vi "CreateClass.vi"(0 "ClassWriterGOOP300.lvclass":refnum<class "ClassWriterGOOP300.lvclass">, 1 "ProjectTreePosition(String or Project Item Ref)":variant, 2 "CreateClassData":T1, 5 "error in (no error)":errorcluster, 6 "KeepLvClassRefOpen(False)":bool, 7 "HeaderToApply (take from VIRef or /use 2D-8bit header, Ignored if not wired)":variant) -> (14 "ClassWriterGOOP300.lvclass":refnum<class "ClassWriterGOOP300.lvclass">, 15 "LVClassLibraryRefnum":refnum<vi>, 16 "TemplateVersionUsed":string, 19 "error out":errorcluster)   [LabVIEW 2020, in "ClassWriterGOOP300.lvclass"]
uses:
  <resource>/Framework/Providers/Open_GDS/ClassProviders/Provider_EndevoGOOP300/ClassWriterGOOP300_class/ClassWriterGOOP300.lvclass
  <resource>/Framework/Providers/Open_GDS/ClassProviders/Provider_BaseClassInterface/CreateClassData.ctl
  <resource>/Framework/Providers/Open_GDS/ClassProviders/Common/LvClass_class/GDSLvCLass_ClassSettingsType.ctl
  <resource>/Framework/Providers/Open_GDS/ClassProviders/Common/LvClass_class/GDSLvClass_PlugIn.ctl
  <resource>/Framework/Providers/Open_GDS/ClassProviders/Common/LvClass_class/GDSLvClass_PlugInTypes.ctl
  <resource>/Framework/Providers/Open_GDS/ClassProviders/Provider_EndevoGOOP400/EndevoG4ProviderName.ctl
  <resource>/Framework/Providers/Open_GDS/ClassProviders/Provider_EndevoGOOP300/EndevoProviderName.ctl
  <resource>/Framework/Providers/Open_GDS/ClassProviders/Provider_BaseClassInterface/ClassWriter_class/ClassWriter.lvclass
  <resource>/Framework/Providers/Open_GDS/ClassProviders/Provider_LvNativeClass/ClassWriterNative_class/ClassWriterNative.lvclass
  <resource>/Framework/Providers/Open_GDS/ClassProviders/Provider_EndevoGOOP400/ClassWriterGOOP400_class/ClassWriterGOOP400.lvclass
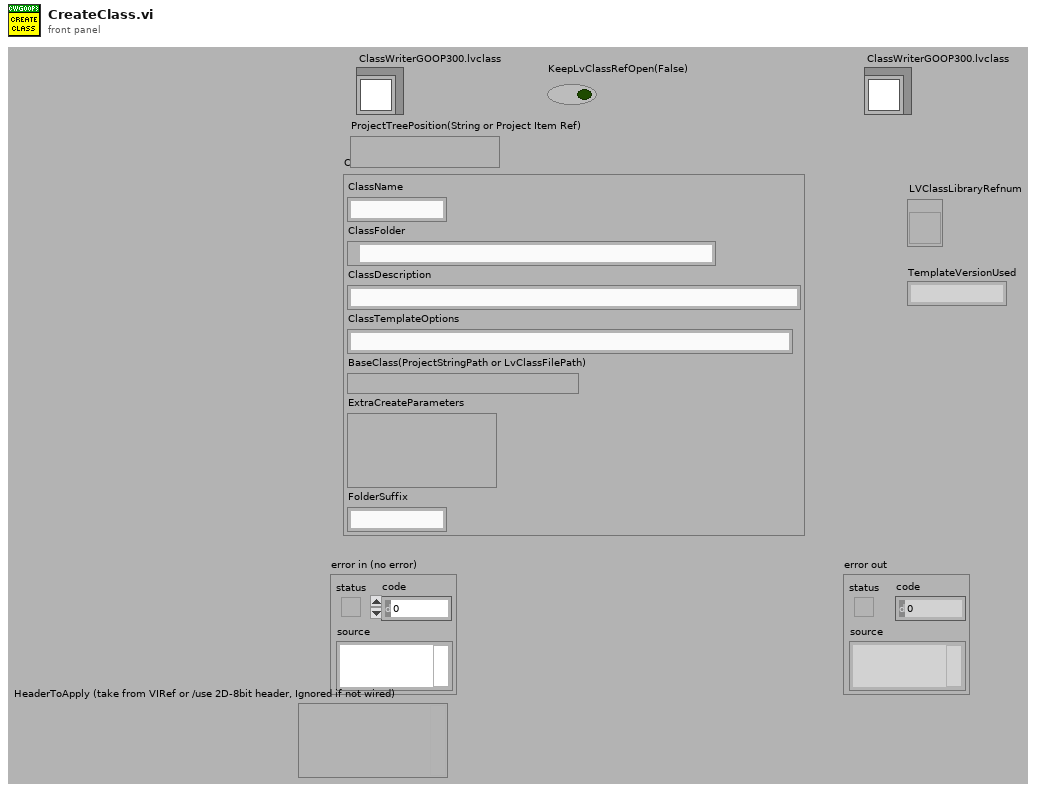
[diagram p1: front panel]
types:
  T1 = typedef "ClassWriter.lvclass/CreateClassData.ctl" = cluster{"ClassName":string, "ClassFolder":path, "ClassDescription":string, "ClassTemplateOptions":string, "BaseClass(ProjectStringPath or LvClassFilePath)":variant, "ExtraCreateParameters":variant, "FolderSuffix":string}
  T2 = typedef "GDSLvCLass_ClassSettingsType.ctl" = cluster{"ClassProviderName":string, "ClassTemplateUsed":string, "ClassTemplateVersion":string, "ClassDescription":string, "PlugIns":T3[], "ConnectorPanePattern":string}
  T3 = typedef "GDSLvClass_PlugIn.ctl" = cluster{"Type":T4, "ID":string, "Version":string, "Path":path, "Name":string, "Data":variant}
  T4 = typedef "GDSLvClass_PlugInTypes.ctl" = enum16{"DesignPattern", "MethodTypes"}
  T5 = cluster{"SubClass":bool, "ClassTemplateFiles":path[], "ClassName":string, "ClassFolder":path, "VIs":refnum<vi>[], "TemplateFolder":path, "ViSubDirs":string[], "TemplateName":string, "BaseClassFolder":path, "RootBaseClassFolder":path, "LvClassPath":path, "ClassRefnum":refnum<vi>, "ProjectRefnum":refnum<vi>, "LvClassFolderPath":path, "BaseClassName":string, "ClassItems":refnum<vi>[], "ViLocked":bool[], "ProjectItemOwner":refnum<vi>, "DeleteFiles":path[], "VIsBefore":refnum<vi>[], "BaseClassPath":path, "BaseConstructorBase":path, "TemplBaseConstructorBase":path, "TemplatePath":path, "TemplateVersion":string, "TemplateParentClass":refnum<vi>, "App":refnum<vi>, "Parent Class":refnum<vi>, "ParentVIs":refnum<vi>[], "TempClass":refnum<vi>, "TemplateParentName":string, "llb":bool, "ClassSettings":T2}
  T6 = typedef "EndevoG4ProviderName.ctl" = enum16{"EndevoGOOP400"}
  T7 = typedef "EndevoProviderName.ctl" = enum16{"EndevoGOOP300"}
  T8 = enum32{"invalid scope", "public", "private", "protected"}
  T9 = enum16{"Share clones between instances", "Preallocate clone for each instance"}
  T10 = enum32{"invalid lock state", "Not Locked", "Locked (No Password)", "Password-protected"}
  T11 = typedef "ClassWriter.lvclass/TemplateSettings.ctl" = cluster{"CommonClassTemplate":bool, "DynamicDispatch":enum8{"False", "True", "Mixed"}, "MustOverride":enum8{"False", "True", "Mixed"}, "MustCallParent":enum8{"False", "True", "Mixed"}, "OnlyNormalMethod":bool, "OnlyPublic":bool}
  T12 = typedef "Scripting_ConnectorPanePatternType.ctl" = u16
  T13 = typedef "GOOP400_Options.ctl" = cluster{"FlatFolderStructure":bool}
  T14 = typedef "imagedata.ctl" = cluster{"image type":i32, "image depth":i32, "image":u8[], "mask":u8[], "colors":u32[], "Rectangle":cluster{"left":i16, "top":i16, "right":i16, "bottom":i16}}
  T15 = typedef "Librarian File Info Out.ctl" = cluster{"creation date":u32, "last mod date":u32, "type":string, "creator":string, "LV version":i32, "size":i32, "top level":bool}
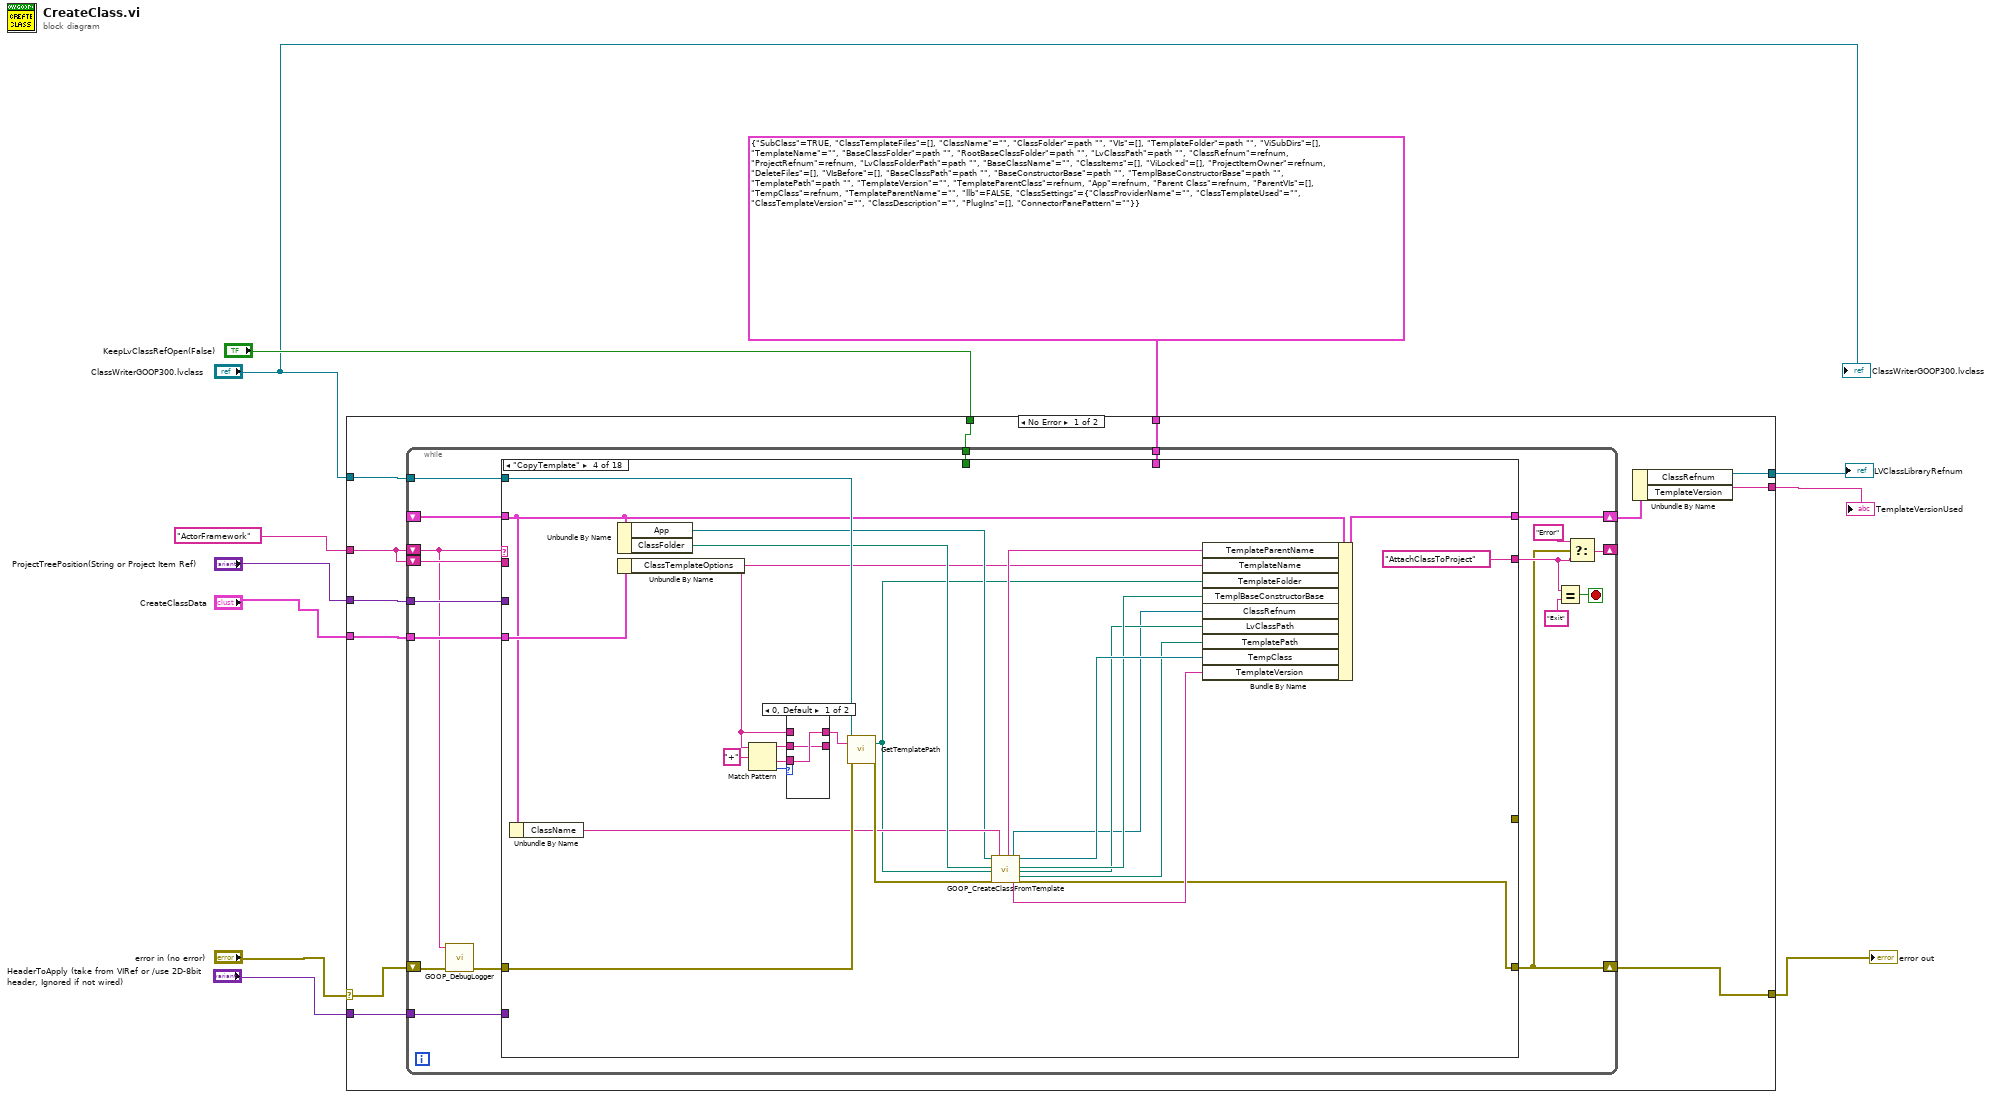
[diagram p0: block diagram]
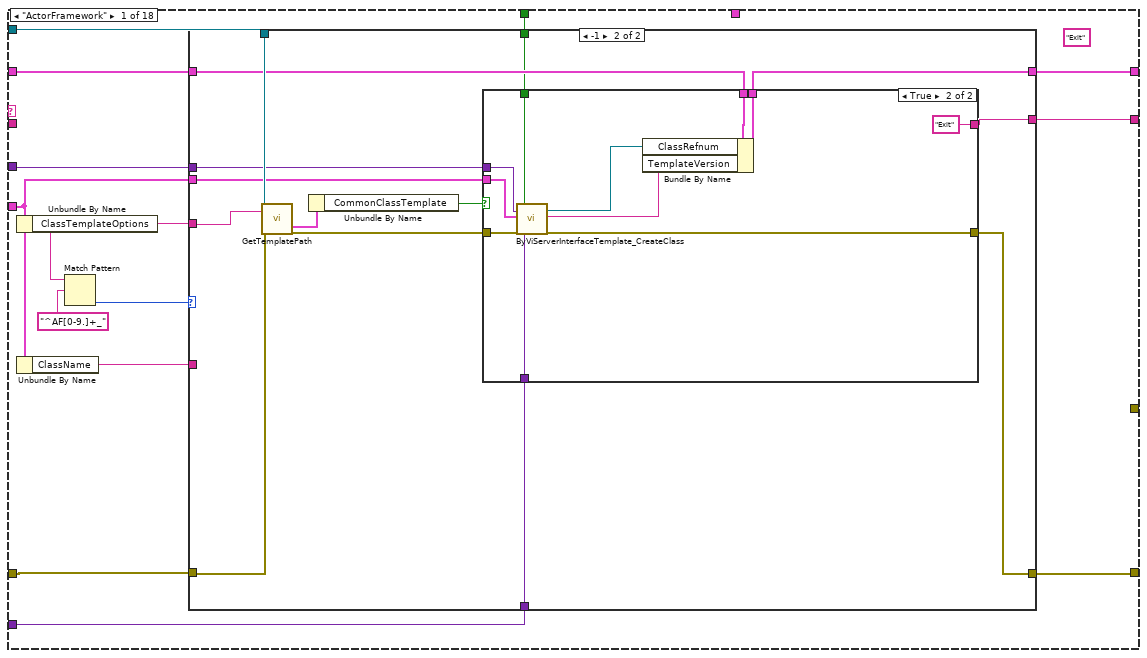
[diagram p2: hidden frame]
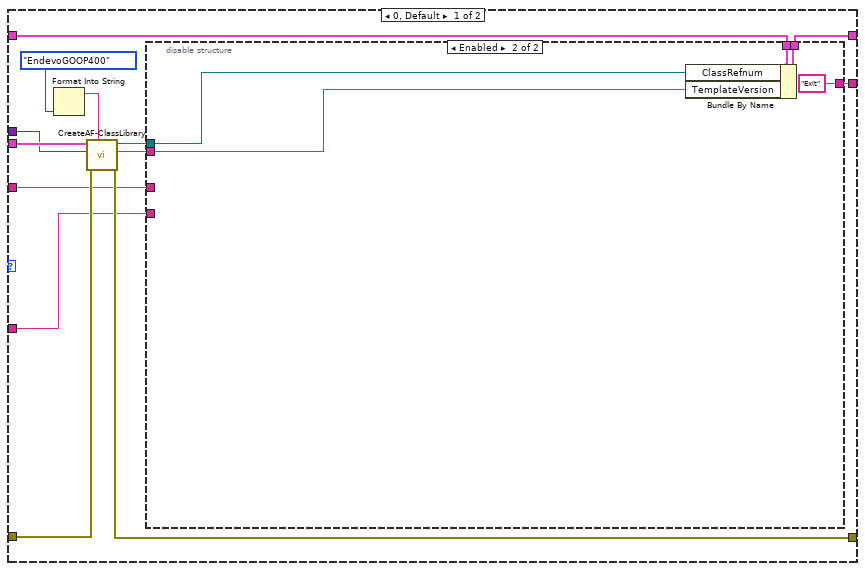
[diagram p3: hidden frame]
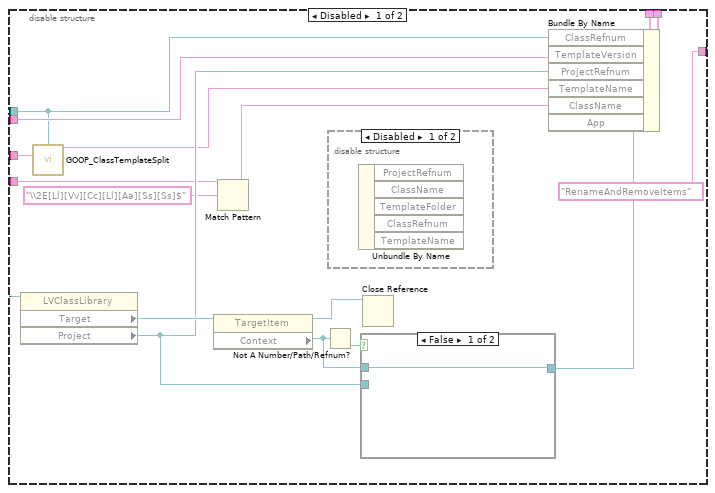
[diagram p4: hidden frame]
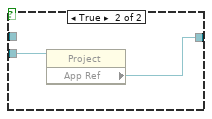
[diagram p6: hidden frame]
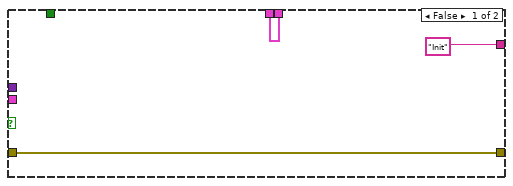
[diagram p7: hidden frame]
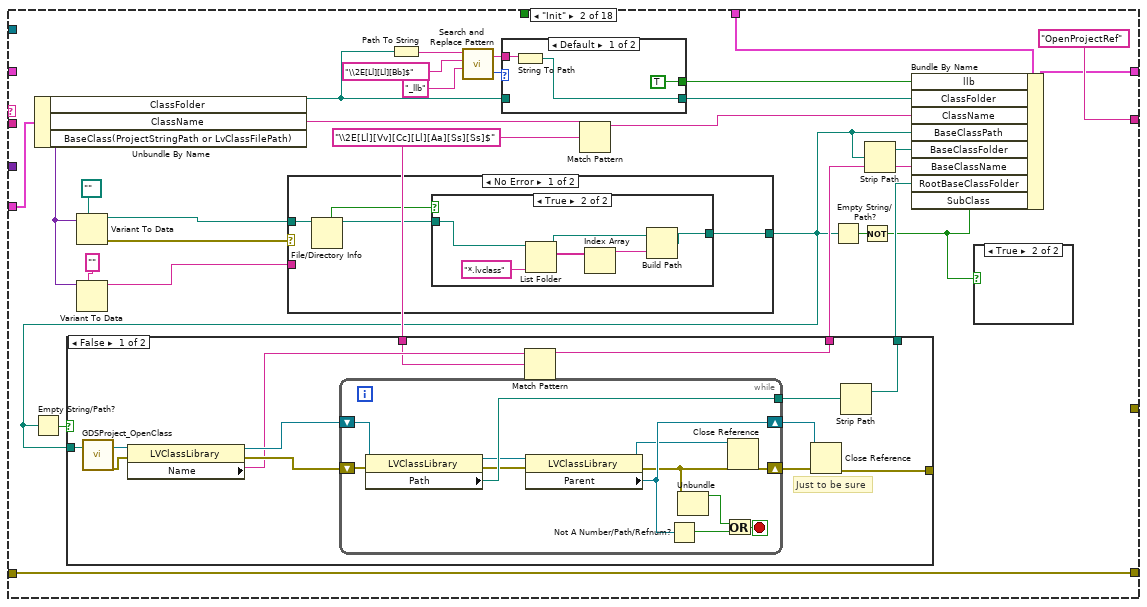
[diagram p8: hidden frame]
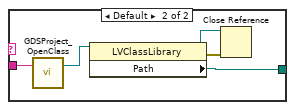
[diagram p14: hidden frame]
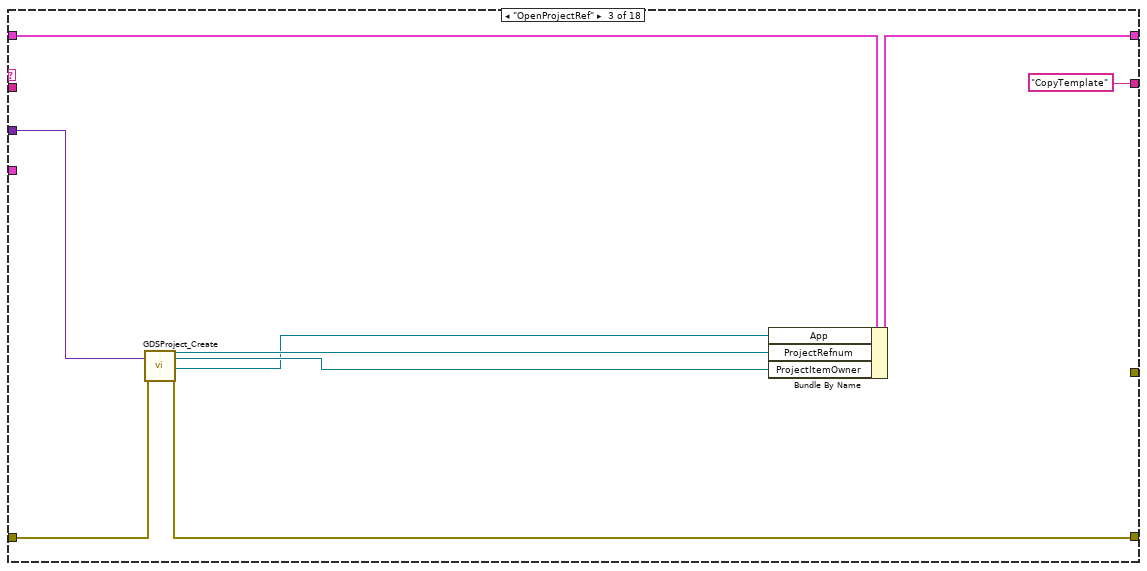
[diagram p15: hidden frame]
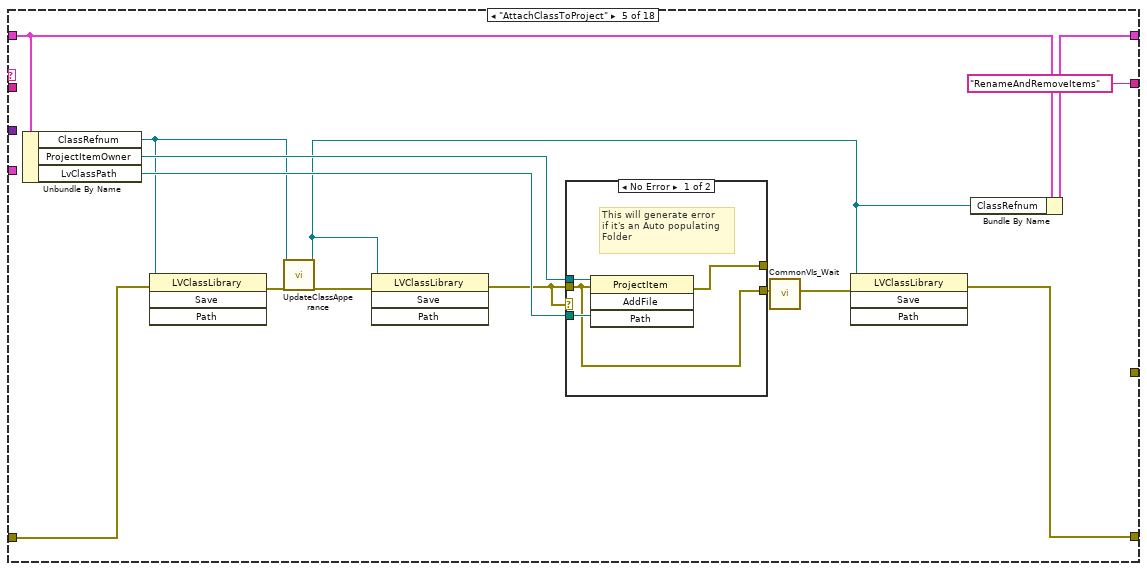
[diagram p17: hidden frame]
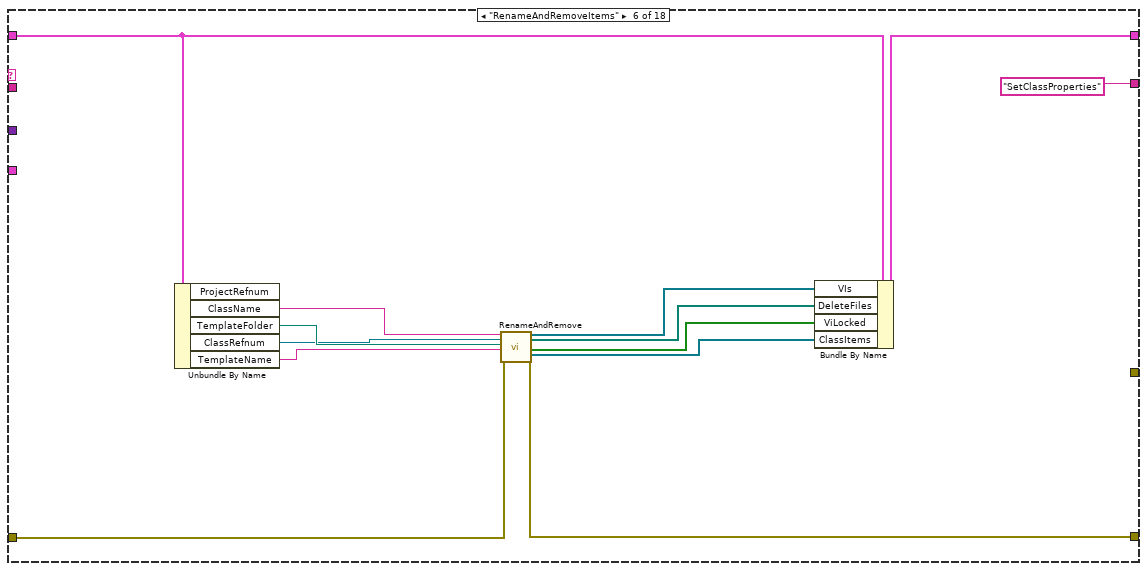
[diagram p19: hidden frame]
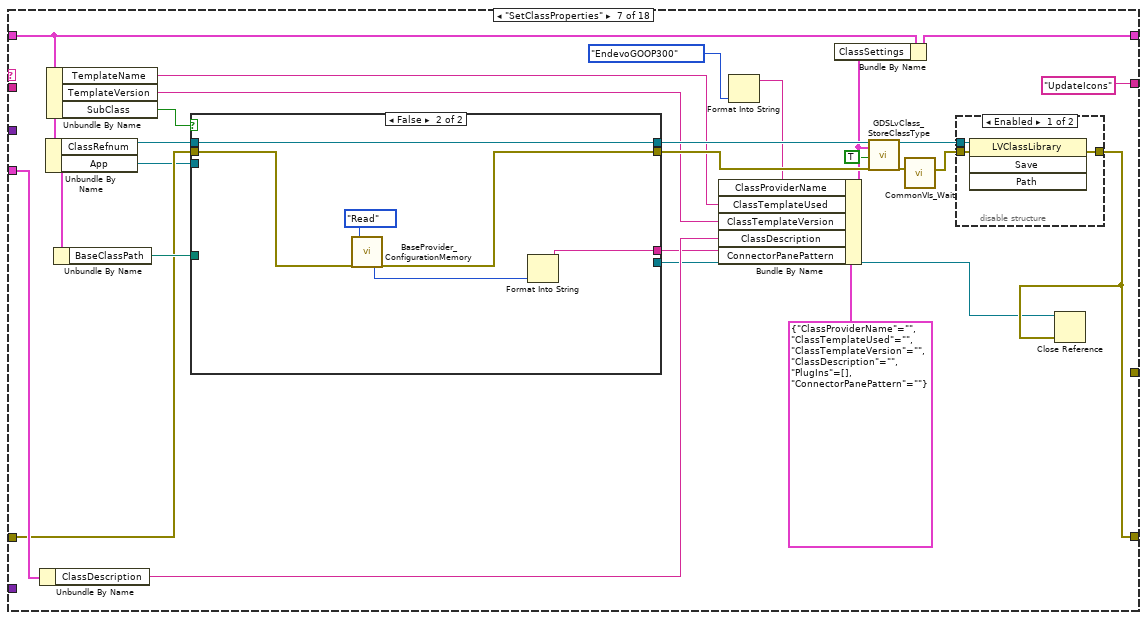
[diagram p20: hidden frame]
diagram:
  n1 = case shown="No Error" "error in (no error)" {
    selector: "error in (no error)" -> [w13 w816]
    tunnel: [w23 w816] -> w11
    tunnel: "ProjectTreePosition(String or Project Item Ref)" -> [w22 _]
    tunnel: "CreateClassData" -> [w21 _]
    tunnel: "ClassWriterGOOP300.lvclass" -> [w20 _]
    tunnel: "HeaderToApply (take from VIRef or /use 2D-8bit header, Ignored if not wired)" -> [w19 _]
    tunnel: "KeepLvClassRefOpen(False)" -> [w18 _]
    tunnel: [w17 _] -> w5
    tunnel: [w16 _] -> w4
    tunnel: T5 {"SubClass"=TRUE, "ClassTemplateFiles"=[], "ClassName"="", "ClassFolder"=path "", "VIs"=[], "TemplateFolder"=path "", "ViSubDirs"=[], "TemplateName"="", "BaseClassFolder"=path "", "RootBaseClassFolder"=path "", "LvClassPath"=path "", "ClassRefnum"=refnum, "ProjectRefnum"=refnum, "LvClassFolderPath"=path "", "BaseClassName"="", "ClassItems"=[], "ViLocked"=[], "ProjectItemOwner"=refnum, "DeleteFiles"=[], "VIsBefore"=[], "BaseClassPath"=path "", "BaseConstructorBase"=path "", "TemplBaseConstructorBase"=path "", "TemplatePath"=path "", "TemplateVersion"="", "TemplateParentClass"=refnum, "App"=refnum, "Parent Class"=refnum, "ParentVIs"=[], "TempClass"=refnum, "TemplateParentName"="", "llb"=FALSE, "ClassSettings"={"ClassProviderName"="", "ClassTemplateUsed"="", "ClassTemplateVersion"="", "ClassDescription"="", "PlugIns"=[], "ConnectorPanePattern"=""}} ("output cluster") -> [w15 _]
    tunnel: "ActorFramework" -> [w12 _]
    frame No Error {
      n2 = while {
        shift-right: [w33] -> w23
        shift-left: w13 -> [w26]
        shift-right: [w37] -> _
        shift-left: w12 -> [w24]
        shift-right: [w40] -> w14
        shift-left: _ -> [w41]
        tunnel: w15 -> [w35]
        tunnel: w22 -> [w32]
        tunnel: w21 -> [w31]
        tunnel: w20 -> [w30]
        shift-left: w12 -> [w29]
        tunnel: w19 -> [w28]
        tunnel: w18 -> [w27]
        stop <- w38 stop-if-true
        n3 = call <resource>:"GOOP_DebugLogger.vi"("error in (no error)"=w26, "State"=w24) -> ("error out"=w25:errorcluster)  [unwired: 7 in, 2 out]
        n4 = case shown="\"CopyTemplate\"" w24 {
          selector: w24 -> [_ _ _ _ _ _ _ _ _ _ _ _ _ _ _ _ _ w767]
          tunnel: w41 -> [w55 _ w203 w214 w245 w260 w278 w328 w350 w364 w497 w550 w583 w635 w661 w672 w720 w751]
          tunnel: [w54 w146 w202 w213 w244 w262 w267 w328 w351 w364 w497 w550 w583 w635 w661 w672 w720 w751] -> w40
          tunnel: w25 -> [w50 w149 w201 w226 w239 w257 w279 w321 w347 w376 w518 w564 w584 w639 w660 w673 w723 w768]
          tunnel: [w49 w149 w199 w211 w235 w258 w270 w318 w333 w362 w498 w565 w585 w640 w659 w673 w706 w764] -> w33
          tunnel: [w53 "OpenProjectRef" "CopyTemplate" "AttachClassToProject" "RenameAndRemoveItems" "SetClassProperties" "UpdateIcons" w330 "UpdateVIs" ("t") "AddFolders" "AddFolders" w549 "PlaceRefInAttribute" "PlaceRefInAttribute" "ReentrantDestructor?" w677 "CloseRefs" "Exit"] -> w34
          tunnel: w35 -> [_ w142 _ _ _ _ _ _ _ _ _ _ _ _ _ _ _ _]
          tunnel: w32 -> [w48 _ w200 _ _ _ _ _ _ _ _ _ _ _ _ _ _ _]
          tunnel: w31 -> [w46 w141 _ w228 _ _ w285 _ _ _ _ _ _ _ _ _ w725 _]
          tunnel: w30 -> [w44 _ _ w227 _ _ _ w315 _ _ _ _ _ w641 _ _ _ _]
          tunnel: w29 -> [_ _ _ _ _ _ _ _ _ _ _ _ _ _ _ _ _ w763]
          tunnel: w28 -> [w42 _ _ _ _ _ _ w326 _ _ _ _ _ _ _ _ _ _]
          tunnel: w27 -> [w43 _ _ _ _ _ _ _ _ _ _ _ _ _ _ _ _ w759]
          tunnel: [_ _ _ _ _ _ _ _ _ _ _ _ _ _ _ _ _ w757] -> _
          frame "ActorFramework" {
            (unwired) "Exit"
            n5 = Unbundle By Name(w46) -> ("ClassTemplateOptions"=w47:string)
            n6 = Unbundle By Name(w46) -> ("ClassName"=w45:string)
            n7 = Match Pattern(string=w47, regular expression="^AF[0-9.]+_") -> (offset past match=w51:i32)  [unwired: 1 in, 3 out]
            n8 = case shown="-1" w51 {
              tunnel: w55 -> [w68 w100]
              tunnel: [w67 w99] -> w54
              tunnel: [w59 w106] -> w53
              tunnel: w46 -> [w65 w96]
              tunnel: w50 -> [w64 w104]
              tunnel: [w63 w101] -> w49
              tunnel: w48 -> [w60 w97]
              tunnel: w47 -> [w57 w103]
              tunnel: w45 -> [w56 _]
              tunnel: w44 -> [_ w105]
              tunnel: w43 -> [_ w98]
              tunnel: w42 -> [_ w95]
              frame 0, Default {
                n9 = Format Into String(EndevoG4ProviderName."EndevoGOOP400" ("ProviderName")) -> (resulting string=w62:string)  [unwired: 3 in, 1 out]
                n10 = call <resource>:"CreateAF-ClassLibrary.vi"("Providername"=w62, "error in (no error)"=w64, "ProjectTreePosition(String or Project Item Ref)"=w60, "CreateClassData"=w65) -> ("error out"=w63:errorcluster, "TemplateVersionUsed"=w61:string, "LVClassLibraryRefnum"=w58:refnum<vi>)  [unwired: 5 in]
                n11 = disable-structure shown="Enabled" {
                  disable-tunnel: w68 -> [w84 w92]
                  disable-tunnel: [w83 w91] -> w67
                  disable-tunnel: w61 -> [w82 w89]
                  disable-tunnel: ["RenameAndRemoveItems" "Exit"] -> w59
                  disable-tunnel: w58 -> [w74 w90]
                  disable-tunnel: w57 -> [w73 _]
                  disable-tunnel: w56 -> [w70 _]
                  frame Disabled {
                    n12 = property class="LVClassLibrary"(reference=w74) -> ("Target"=w80:refnum<vi>, "Project"=w75:refnum<vi>)  [unwired: 1 in, 2 out]
                    n13 = call <resource>:"GOOP_ClassTemplateSplit.vi"("ClassItemRefIn"=w74, "FullClassTemplate"=w73) -> ("StandardTemplate"=w72:string)  [unwired: 12 in, 1 out]
                    n14 = property class="TargetItem"(reference=w80) -> (reference out=w79:refnum<vi>, "Context"=w77:refnum<vi>)  [unwired: 1 in, 1 out]
                    n15 = Match Pattern(string=w70, regular expression="\\2E[Ll][Vv][Cc][Ll][Aa][Ss][Ss]$") -> (before substring=w69:string)  [unwired: 1 in, 3 out]
                    n16 = Not A Number/Path/Refnum?(number/path/refnum=w77) -> (NaN/Path/Refnum?=w78:bool)
                    n17 = disable-structure shown="Disabled" {
                      frame Disabled {
                        n18 = Unbundle By Name() -> ()  [unwired: 1 in, 5 out]
                      }
                      frame Enabled {
                      }
                    }
                    n19 = case shown="False" w78 {
                      tunnel: [w85 w86] -> w76
                      tunnel: w75 -> [_ w87]
                      tunnel: w77 -> [w85 _]
                      frame False {
                      }
                      frame True {
                        n20 = property class="Project"(reference=w87) -> ("App Ref"=w86:refnum<vi>)  [unwired: 1 in, 2 out]
                      }
                    }
                    n21 = Close Reference(reference=w79) -> ()  [unwired: 1 in, 1 out]
                    n22 = Bundle By Name(cluster=w84, "ClassRefnum"=w74, "TemplateVersion"=w82, "ProjectRefnum"=w75, "TemplateName"=w72, "ClassName"=w69, "App"=w76) -> (w83:T5)
                  }
                  frame Enabled {
                    n23 = Bundle By Name(cluster=w92, "ClassRefnum"=w90, "TemplateVersion"=w89) -> (w91:T5)
                  }
                }
              }
              frame -1 {
                n24 = call-dynamic "GetTemplatePath.vi"("reference in"=w105, "ClassTemplateSubDirectory"=w103, "error in (no error)"=w104) -> ("TemplateSettings"=w94:T11, "error out"=w102:errorcluster)  [unwired: 12 in, 3 out]
                n25 = Unbundle By Name(w94) -> ("CommonClassTemplate"=w93:bool)
                n26 = case shown="True" w93 {
                  tunnel: ["Init" "Exit"] -> w106
                  tunnel: w102 -> [w107 w117]
                  tunnel: [w107 w116] -> w101
                  tunnel: w100 -> [w108 w115]
                  tunnel: [w108 w114] -> w99
                  tunnel: w98 -> [_ w113]
                  tunnel: w97 -> [_ w112]
                  tunnel: w96 -> [_ w111]
                  tunnel: w95 -> [_ w110]
                  frame False {
                  }
                  frame True {
                    n27 = call <resource>:"ByViServerInterfaceTemplate_CreateClass.vi"("ProjectTreePosition(String or Project Item Ref)"=w112, "CreateClassData"=w111, "error in (no error)"=w117, "KeepLvClassRefOpen(False)"=w113, "HeaderToApply (take from VIRef or /use 2D-8bit header, Ignored if not wired)"=w110) -> ("LVClassLibraryRefnum"=w119:refnum<vi>, "TemplateVersionUsed"=w118:string, "error out"=w116:errorcluster)  [unwired: 12 in]
                    n28 = Bundle By Name(cluster=w115, "ClassRefnum"=w119, "TemplateVersion"=w118) -> (w114:T5)
                  }
                }
              }
            }
          }
          frame "Init" {
            w138 = "\\2E[Ll][Vv][Cc][Ll][Aa][Ss][Ss]$" ("regular expression")
            n29 = Unbundle By Name(w141) -> ("ClassFolder"=w124:path, "ClassName"=w135:string, "BaseClass(ProjectStringPath or LvClassFilePath)"=w140:variant)
            n30 = Variant To Data(type=path "" ("path"), Variant=w140) -> (data=w132:path, error out=w133:errorcluster)  [unwired: 1 in]
            n31 = Variant To Data(type="" ("regular expression"), Variant=w140) -> (data=w143:string)  [unwired: 1 in, 1 out]
            n32 = case shown="No Error" w133 {
              tunnel: [w181 w189] -> w130
              tunnel: w143 -> [_ w190]
              tunnel: w132 -> [w180 _]
              frame No Error {
                n33 = File/Directory Info(path=w180) -> (path out=w178:path, directory=w179:bool)  [unwired: 1 in, 5 out]
                n34 = case shown="True" w179 {
                  tunnel: [w182 w184] -> w181
                  tunnel: w178 -> [w182 w183]
                  frame False {
                  }
                  frame True {
                    n35 = List Folder(path=w183, pattern="*.lvclass") -> (path out=w185:path, filenames=w187:string[])  [unwired: 2 in, 2 out]
                    n36 = Index Array(array=w187) -> (element=w186:string)  [unwired: 1 in]
                    n37 = Build Path(base path=w185, name or relative path=w186) -> (appended path=w184:path)
                  }
                }
              }
              frame Error {
                n38 = case shown="\"\"" w190 {
                  tunnel: w190 -> [_ w195]
                  tunnel: [_ w191] -> w189
                  frame "" {
                  }
                  frame Default {
                    n39 = call <resource>:"GDSProject_OpenClass.vi"("ClassPath(FilePath/ProjectTreePath/LvCLassRef)"=w195) -> ("LVClass.Open"=w194:refnum<vi>)  [unwired: 16 in, 2 out]
                    n40 = property class="LVClassLibrary"(reference=w194) -> (reference out=w192:refnum<vi>, error out=w193:errorcluster, "Path"=w191:path)  [unwired: 1 in]
                    n41 = Close Reference(reference=w192, error in (no error)=w193) -> ()  [unwired: 1 out]
                  }
                }
              }
            }
            n42 = Empty String/Path?(string/path=w130) -> (empty?=w136:bool)
            n43 = case shown="False" w136 {
              tunnel: [w163 _] -> w139
              tunnel: w138 -> [w157 _]
              tunnel: [w156 _] -> w137
              tunnel: w130 -> [w155 _]
              tunnel: [w154 _] -> _
              frame False {
                # "Just to be sure"
                n44 = call <resource>:"GDSProject_OpenClass.vi"("ClassPath(FilePath/ProjectTreePath/LvCLassRef)"=w155) -> ("LVClass.Open"=w160:refnum<vi>, "error out"=w162:errorcluster)  [unwired: 16 in, 1 out]
                n45 = property class="LVClassLibrary"(reference=w160, error in=w162) -> (reference out=w159:refnum<vi>, error out=w161:errorcluster, "Name"=w158:string)
                n46 = while {
                  shift-right: [w174] -> w166
                  shift-left: w161 -> [w169]
                  shift-right: [w175] -> w165
                  shift-left: w159 -> [w177]
                  tunnel: [w176] -> w164
                  stop <- w171 stop-if-true
                  n47 = property class="LVClassLibrary"(reference=w177, error in=w169) -> (reference out=w167:refnum<vi>, error out=w168:errorcluster, "Path"=w176:path)
                  n48 = property class="LVClassLibrary"(reference=w167, error in=w168) -> (reference out=w170:refnum<vi>, error out=w174:errorcluster, "Parent"=w175:refnum<vi>)
                  n49 = Not A Number/Path/Refnum?(number/path/refnum=w175) -> (NaN/Path/Refnum?=w172:bool)
                  n50 = Unbundle(w174) -> ("status"=w173:bool)  [unwired: 2 out]
                  n51 = Or(x=w173, y=w172) -> (x .or. y?=w171:bool)
                  n52 = Close Reference(reference=w170) -> ()  [unwired: 1 in, 1 out]
                }
                n53 = Match Pattern(string=w158, regular expression=w157) -> (before substring=w156:string)  [unwired: 1 in, 3 out]
                n54 = Close Reference(reference=w165, error in (no error)=w166) -> (error out=w154:errorcluster)
                n55 = Strip Path(path=w164) -> (stripped path=w163:path)  [unwired: 1 out]
              }
              frame True {
              }
            }
            n56 = Path To String(path=w124) -> (string=w128:string)
            n57 = call <vilib>:"Search and Replace Pattern.vi"("string"=w128, "regular expression (\"\")"="\\2E[Ll][Ll][Bb]$" ("regular expression (\"\")"), "replace string (\"\")"="_llb" ("replace string (\"\")")) -> ("result string"=w121:string, "offset past match"=w126:i32)  [unwired: 2 in]
            n58 = case shown="Default" w126 {
              tunnel: w124 -> [_ w153]
              tunnel: [w150 w153] -> w123
              tunnel: [TRUE _] -> w122
              tunnel: w121 -> [w151 _]
              frame Default {
                n59 = String To Path(string=w151) -> (path=w150:path)
              }
              frame -1 {
              }
            }
            n60 = Match Pattern(string=w135, regular expression=w138) -> (before substring=w147:string)  [unwired: 1 in, 3 out]
            n61 = Empty String/Path?(string/path=w130) -> (empty?=w131:bool)
            n62 = Not(x=w131) -> (.not. x?=w129:bool)
            n63 = Strip Path(path=w130) -> (stripped path=w134:path)  [unwired: 1 out]
            n64 = Bundle By Name(cluster=w142, "llb"=w122, "ClassFolder"=w123, "ClassName"=w147, "BaseClassPath"=w130, "BaseClassFolder"=w134, "BaseClassName"=w137, "RootBaseClassFolder"=w139, "SubClass"=w129) -> (w146:T5)
            n65 = case shown="True" w129 {
              frame False {
              }
              frame True {
              }
            }
          }
          frame "OpenProjectRef" {
            n66 = call <resource>:"GDSProject_Create.vi"("ProjectTreePosition(String or Project Item Ref)"=w200, "error in (no error)"=w201) -> ("Project Refnum"=w197:refnum<vi>, "Project Item"=w198:refnum<vi>, "App"=w196:refnum<vi>, "error out"=w199:errorcluster)  [unwired: 14 in]
            n67 = Bundle By Name(cluster=w203, "App"=w196, "ProjectRefnum"=w197, "ProjectItemOwner"=w198) -> (w202:T5)
          }
          frame "CopyTemplate" {
            n68 = Unbundle By Name(w214) -> ("ClassName"=w208:string)
            n69 = Unbundle By Name(w214) -> ("App"=w207:refnum<vi>, "ClassFolder"=w209:path)
            n70 = Unbundle By Name(w228) -> ("ClassTemplateOptions"=w206:string)
            n71 = Match Pattern(string=w206, regular expression="+") -> (before substring=w222:string, after substring=w225:string, offset past match=w224:i32)  [unwired: 1 in, 1 out]
            n72 = case shown="0, Default" w224 {
              tunnel: w206 -> [_ w232]
              tunnel: [w231 w232] -> w221
              tunnel: w225 -> [w231 _]
              tunnel: [w230 _] -> _
              tunnel: w222 -> [w230 _]
              frame 0, Default {
              }
              frame -1 {
              }
            }
            n73 = call-dynamic "GetTemplatePath.vi"("reference in"=w227, "ClassTemplateSubDirectory"=w221, "error in (no error)"=w226) -> ("FolderPathOut"=w205:path, "error out"=w210:errorcluster)  [unwired: 12 in, 3 out]
            n74 = call <resource>:"GOOP_CreateClassFromTemplate.vi"("Application in"=w207, "ClassFolder"=w209, "TeplateClassFolder"=w205, "error in (no error)"=w210, "ClassName"=w208) -> ("TemplateParentName"=w212:string, "NewClassRef"=w217:refnum<vi>, "TemplateClassVersionString"=w215:string, "TemplateClassRef"=w220:refnum<vi>, "TemplateClassConstructorPath(*Create, *Init)"=w219:path, "NewClassPath"=w218:path, "TemplateClassPath"=w216:path, "error out"=w211:errorcluster)  [unwired: 7 in]
            n75 = Bundle By Name(cluster=w214, "TemplateParentName"=w212, "TemplateName"=w206, "TemplateFolder"=w205, "TemplBaseConstructorBase"=w219, "ClassRefnum"=w217, "LvClassPath"=w218, "TemplatePath"=w216, "TempClass"=w220, "TemplateVersion"=w215) -> (w213:T5)
          }
          frame "AttachClassToProject" {
            n76 = Unbundle By Name(w245) -> ("ClassRefnum"=w238:refnum<vi>, "ProjectItemOwner"=w246:refnum<vi>, "LvClassPath"=w242:path)
            n77 = invoke class="LVClassLibrary" method="Save"(reference=w238, error in=w239) -> (error out=w240:errorcluster)  [unwired: 2 in, 3 out]
            n78 = call <resource>:"UpdateClassApperance.vi"("ClassRefIn"=w238, "error in (no error)"=w240) -> ("ClassRefOut"=w233:refnum<vi>, "error out"=w237:errorcluster)  [unwired: 16 in]
            n79 = invoke class="LVClassLibrary" method="Save"(reference=w233, error in=w237) -> (error out=w234:errorcluster)  [unwired: 2 in, 3 out]
            n80 = case shown="No Error" w234 {
              tunnel: w246 -> [w250 _]
              tunnel: w242 -> [w249 _]
              tunnel: [w248 w251] -> w241
              tunnel: w234 -> [w248 w251]
              tunnel: [w247 _] -> _
              frame No Error {
                # "This will generate error\nif it's an Auto populating\nFolder"
                n81 = invoke class="ProjectItem" method="AddFile"(reference=w250, error in=w248, "Path"=w249) -> (error out=w247:errorcluster)  [unwired: 1 in, 3 out]
              }
              frame Error {
              }
            }
            n82 = call <resource>:"CommonVIs_Wait.vi"("error in"=w241) -> ("error out"=w236:errorcluster)  [unwired: 9 in]
            n83 = invoke class="LVClassLibrary" method="Save"(reference=w233, error in=w236) -> (error out=w235:errorcluster)  [unwired: 2 in, 3 out]
            n84 = Bundle By Name(cluster=w245, "ClassRefnum"=w233) -> (w244:T5)
          }
          frame "RenameAndRemoveItems" {
            n85 = Unbundle By Name(w260) -> ("ClassName"=w264:string, "TemplateFolder"=w261:path, "ClassRefnum"=w259:refnum<vi>, "TemplateName"=w252:string)  [unwired: 1 out]
            n86 = call <resource>:"RenameAndRemove.vi"("ClassName"=w264, "ClassRefnum"=w259, "TemplateFolder"=w261, "TemplateName"=w252, "error in"=w257) -> ("ViRefsOut"=w263:refnum<vi>[], "DeleteFiles"=w256:path[], "ItemLocked"=w255:bool[], "Items"=w254:refnum<vi>[], "error out"=w258:errorcluster)  [unwired: 10 in]
            n87 = Bundle By Name(cluster=w260, "VIs"=w263, "DeleteFiles"=w256, "ViLocked"=w255, "ClassItems"=w254) -> (w262:T5)
          }
          frame "SetClassProperties" {
            n88 = Unbundle By Name(w285) -> ("ClassDescription"=w282:string)
            n89 = Unbundle By Name(w278) -> ("ClassRefnum"=w280:refnum<vi>, "App"=w275:refnum<vi>)
            n90 = Unbundle By Name(w278) -> ("TemplateName"=w281:string, "TemplateVersion"=w276:string, "SubClass"=w289:bool)
            n91 = Unbundle By Name(w278) -> ("BaseClassPath"=w288:path)
            n92 = case shown="False" w289 {
              tunnel: w280 -> [w297 w314]
              tunnel: [w308 w314] -> w287
              tunnel: w279 -> [w301 w310]
              tunnel: [w307 w309] -> w286
              tunnel: w288 -> [w306 _]
              tunnel: w275 -> [w302 _]
              tunnel: [w303 w311] -> w274
              tunnel: [w295 _] -> w269
              frame True {
                n93 = invoke class="LVClassLibrary" method="Save"(reference=w297) -> (reference out=w296:refnum<vi>)  [unwired: 3 in, 3 out]
                n94 = invoke class="App" method="LVClass.Open"(reference=w302, error in=w301, "Path"=w306) -> (error out=w300:errorcluster, "LVClass.Open"=w305:refnum<vi>)  [unwired: 1 in, 2 out]
                n95 = call <resource>:"CommonVIs_Wait.vi"("error in"=w300) -> ("error out"=w299:errorcluster)  [unwired: 9 in]
                n96 = call <resource>:"GDSLvClass_ReadClassType.vi"("Class Refnum In"=w305, "error in (no error)"=w299) -> ("Class Refnum Out"=w295:refnum<vi>, "ClassSettings"=w304:T2, "error out"=w298:errorcluster)  [unwired: 15 in]
                n97 = Unbundle By Name(w304) -> ("ConnectorPanePattern"=w303:string)
                n98 = invoke class="LVClassLibrary" method="Save"(reference=w295) -> (reference out=w294:refnum<vi>)  [unwired: 3 in, 3 out]
                n99 = property class="LVClassLibrary"(reference=w296, error in=w298, "Parent"=w294) -> (reference out=w308:refnum<vi>, error out=w307:errorcluster)
              }
              frame False {
                n100 = call <resource>:"BaseProvider_ConfigurationMemory.vi"("error in (no error)"=w310, "Action"=enum16{"Read", "Load", "Save"}."Read") -> ("PatternOut"=w313:T12, "error out"=w309:errorcluster)  [unwired: 11 in, 5 out]
                n101 = Format Into String(w313) -> (resulting string=w311:string)  [unwired: 3 in, 1 out]
              }
            }
            n102 = Format Into String(EndevoProviderName."EndevoGOOP300" ("ProviderName")) -> (resulting string=w283:string)  [unwired: 3 in, 1 out]
            n103 = Bundle By Name(cluster=T2 {"ClassProviderName"="", "ClassTemplateUsed"="", "ClassTemplateVersion"="", "ClassDescription"="", "PlugIns"=[], "ConnectorPanePattern"=""} ("ClassSettings"), "ClassProviderName"=w283, "ClassTemplateUsed"=w281, "ClassTemplateVersion"=w276, "ClassDescription"=w282, "ConnectorPanePattern"=w274) -> (w266:T2)
            n104 = Bundle By Name(cluster=w278, "ClassSettings"=w266) -> (w267:T5)
            n105 = call <resource>:"GDSLvClass_StoreClassType.vi"("Class Refnum In"=w287, "ClassSettings"=w266, "CheckAndFixConnectorPaneType(False)"=TRUE, "error in (no error)"=w286) -> ("Class Refnum Out"=w273:refnum<vi>, "error out"=w272:errorcluster)  [unwired: 14 in]
            n106 = call <resource>:"CommonVIs_Wait.vi"("error in"=w272) -> ("error out"=w271:errorcluster)  [unwired: 9 in]
            n107 = disable-structure shown="Enabled" {
              disable-tunnel: [w292 w293] -> w270
              disable-tunnel: w273 -> [w291 _]
              disable-tunnel: w271 -> [w290 w293]
              frame Enabled {
                n108 = invoke class="LVClassLibrary" method="Save"(reference=w291, error in=w290) -> (error out=w292:errorcluster)  [unwired: 2 in, 3 out]
              }
              frame Disabled {
              }
            }
            n109 = Close Reference(reference=w269, error in (no error)=w270) -> ()  [unwired: 1 out]
          }
          frame "UpdateIcons" {
            n110 = Unbundle By Name(w328) -> ("ClassRefnum"=w327:refnum<vi>)
            n111 = Unbundle By Name(w328) -> ("SubClass"=w332:bool, "ClassName"=w329:string)
            n112 = call-dynamic "ProgressWindow.vi"("ClassWriter in"=w315, "Message(Exit)"="Hide", "error in (no error)"=w321) -> ("ClassWriter out"=w316:refnum<class "ClassWriterGOOP300.lvclass">, "error out"=w320:errorcluster)  [unwired: 15 in]
            n113 = Empty String/Path?(string/path=w326) -> (empty?=w325:bool)
            n114 = Not(x=w325) -> (.not. x?=w324:bool)
            n115 = call <resource>:"GDSLvIcon_DialogUpdateClass.vi"("ClassPath(FilePath/ProjectTreePath/LvCLassRef)"=w327, "ClassName"=w329, "AutoUpdate"=w324, "error in (no error)"=w320, "HeaderToApply (take from VIRef or /use 2D-8bit header, Ignored if not wired)"=w326) -> ("error out"=w319:errorcluster)  [unwired: 11 in, 3 out]
            n116 = Select(t="GetDerivedClassConstructor", s=w332, f="AddFolders") -> (s? t:f=w330:string)
            n117 = call-dynamic "ProgressWindow.vi"("ClassWriter in"=w316, "Message(Exit)"="UnHide", "error in (no error)"=w319) -> ("error out"=w318:errorcluster)  [unwired: 15 in, 1 out]
          }
          frame "GetDerivedClassConstructor" {
            # "USE BASE CLASS PATH"
            n118 = Unbundle By Name(w350) -> ("ClassRefnum"=w348:refnum<vi>)
            n119 = property class="LVClassLibrary"(reference=w348, error in=w347) -> (error out=w344:errorcluster, "Parent"=w336:refnum<vi>)  [unwired: 1 out]
            n120 = property class="LVClassLibrary"(reference=w336, error in=w344) -> (reference out=w335:refnum<vi>, error out=w334:errorcluster, "Path"=w342:path)
            n121 = Strip Path(path=w342) -> (stripped path=w341:path)  [unwired: 1 out]
            n122 = call <vilib>:"Recursive File List.vi"("pattern"="*_Create.vi", "Treat LLBs as Folders?"=TRUE, "Folder Path"=w341) -> ("All Files in Dir"=w339:path[], "dup Folder Path"=w337:path)  [unwired: 4 in, 3 out]
            n123 = Close Reference(reference=w335, error in (no error)=w334) -> (error out=w333:errorcluster)
            n124 = Array Size(array=w339) -> (size(s)=w340:i32)
            n125 = case shown="0" w340 {
              tunnel: w339 -> [w352 _]
              tunnel: [w352 w353] -> w338
              tunnel: w337 -> [_ w354]
              frame Default {
              }
              frame 0 {
                n126 = call <vilib>:"Recursive File List.vi"("pattern"="*_Init.vi", "Treat LLBs as Folders?"=TRUE, "Folder Path"=w354) -> ("All Files in Dir"=w353:path[])  [unwired: 4 in, 4 out]
              }
            }
            n127 = Index Array(array=w338) -> (element=w343:path)  [unwired: 1 in]
            n128 = Bundle By Name(cluster=w350, "BaseConstructorBase"=w343) -> (w351:T5)
          }
          frame "UpdateVIs" {
            (unwired) "AnyProtectedAttributesToUpdate?"
            # "This is a sub class, replace all BaseClass References with Select base class.\nIf base not equal to root, also replace BaseClass ObjectRef with Root-Base ObjectRef"
            n129 = Unbundle By Name(w364) -> ("TemplBaseConstructorBase"=w361:path, "BaseConstructorBase"=w357:path)
            n130 = Unbundle By Name(w364) -> ("VIs"=w377:refnum<vi>[])
            n131 = call <resource>:"CreateVINamesToReplace.vi"("Foldername"="utils" ("name or relative path"), "NewVIName"="_New.vi" ("string"), "BaseConstructorBase"=w357, "TemplBaseConstructorBase"=w361) -> ("NewVIName"=w372:path, "OldVIName"=w373:path)  [unwired: 5 in]
            n132 = call <resource>:"CreateVINamesToReplace.vi"("NewVIName"="_Init.vi" ("string"), "BaseConstructorBase"=w357, "TemplBaseConstructorBase"=w361) -> ("NewVIName"=w368:path, "OldVIName"=w369:path)  [unwired: 6 in]
            n133 = call <resource>:"CreateVINamesToReplace.vi"("NewVIName"="_CleanUp.vi" ("string"), "BaseConstructorBase"=w357, "TemplBaseConstructorBase"=w361) -> ("NewVIName"=w365:path, "OldVIName"=w366:path)  [unwired: 6 in]
            n134 = call <resource>:"CreateVINamesToReplace.vi"("NewVIName"="_GOOPKernel.vi" ("string"), "BaseConstructorBase"=w357, "TemplBaseConstructorBase"=w361) -> ("NewVIName"=w358:path, "OldVIName"=w359:path)  [unwired: 6 in]
            n135 = for {
              shift-right: [w408] -> w362
              shift-left: w376 -> [w405]
              tunnel: w377 -> [w399] mode=indexing
              tunnel: w361 -> [w407]
              tunnel: w357 -> [w406]
              tunnel: w373 -> [w398]
              tunnel: w372 -> [w397]
              tunnel: w369 -> [w391]
              tunnel: w368 -> [w390]
              tunnel: w366 -> [w386]
              tunnel: w365 -> [w385]
              tunnel: w359 -> [w384]
              tunnel: w358 -> [w383]
              n136 = property class="VI"(reference=w399) -> ("Name"=w380:string)  [unwired: 1 in, 2 out]
              n137 = Match Pattern(string=w380, regular expression="_Create.vi") -> (offset past match=w404:i32)  [unwired: 1 in, 3 out]
              n138 = Match Pattern(string=w380, regular expression="_New.vi") -> (offset past match=w402:i32)  [unwired: 1 in, 3 out]
              n139 = Match Pattern(string=w380, regular expression="_Init.vi") -> (offset past match=w395:i32)  [unwired: 1 in, 3 out]
              n140 = Match Pattern(string=w380, regular expression="_CleanUp.vi") -> (offset past match=w388:i32)  [unwired: 1 in, 3 out]
              n141 = Match Pattern(string=w380, regular expression="_GOOPKernel.vi") -> (offset past match=w382:i32)  [unwired: 1 in, 3 out]
              n142 = Greater Or Equal To 0?(x=w404) -> (x >= 0?=w393:bool)
              n143 = Greater Or Equal To 0?(x=w402) -> (x >= 0?=w401:bool)
              n144 = Greater Or Equal To 0?(x=w395) -> (x >= 0?=w392:bool)
              n145 = Greater Or Equal To 0?(x=w388) -> (x >= 0?=w387:bool)
              n146 = Greater Or Equal To 0?(x=w382) -> (x >= 0?=w379:bool)
              n147 = Compound Arithmetic op=OR(w393, w401, w392, w387, w379) -> (w400:bool)
              n148 = case shown="True" w400 {
                tunnel: w405 -> [w409 w428]
                tunnel: [w409 w427] -> w408
                tunnel: w399 -> [_ w426]
                tunnel: w407 -> [_ w424]
                tunnel: w406 -> [_ w423]
                tunnel: w401 -> [_ w425]
                tunnel: w398 -> [_ w420]
                tunnel: w397 -> [_ w419]
                tunnel: w392 -> [_ w418]
                tunnel: w391 -> [_ w417]
                tunnel: w390 -> [_ w416]
                tunnel: w387 -> [_ w415]
                tunnel: w386 -> [_ w414]
                tunnel: w385 -> [_ w413]
                tunnel: w384 -> [_ w412]
                tunnel: w383 -> [_ w411]
                tunnel: w379 -> [_ w410]
                frame False {
                }
                frame True {
                  n149 = case shown="False" w425 {
                    tunnel: w424 -> [w440 _]
                    tunnel: w423 -> [w438 _]
                    tunnel: [w439 w468] -> w422
                    tunnel: [w437 w467] -> w421
                    tunnel: w420 -> [_ w468]
                    tunnel: w419 -> [_ w467]
                    tunnel: w418 -> [w441 _]
                    tunnel: w417 -> [w436 _]
                    tunnel: w416 -> [w435 _]
                    tunnel: w415 -> [w434 _]
                    tunnel: w414 -> [w433 _]
                    tunnel: w413 -> [w432 _]
                    tunnel: w412 -> [w431 _]
                    tunnel: w411 -> [w430 _]
                    tunnel: w410 -> [w429 _]
                    frame False {
                      n150 = case shown="False" w441 {
                        tunnel: w440 -> [w450 _]
                        tunnel: [w447 w466] -> w439
                        tunnel: w438 -> [w448 _]
                        tunnel: [w449 w465] -> w437
                        tunnel: w436 -> [_ w466]
                        tunnel: w435 -> [_ w465]
                        tunnel: w434 -> [w451 _]
                        tunnel: w433 -> [w446 _]
                        tunnel: w432 -> [w445 _]
                        tunnel: w431 -> [w444 _]
                        tunnel: w430 -> [w443 _]
                        tunnel: w429 -> [w442 _]
                        frame False {
                          n151 = case shown="False" w451 {
                            tunnel: [w457 w464] -> w447
                            tunnel: w450 -> [w458 _]
                            tunnel: [w456 w463] -> w449
                            tunnel: w448 -> [w455 _]
                            tunnel: w446 -> [_ w464]
                            tunnel: w445 -> [_ w463]
                            tunnel: w444 -> [w454 _]
                            tunnel: w443 -> [w453 _]
                            tunnel: w442 -> [w452 _]
                            frame False {
                              n152 = case shown="True" w452 {
                                tunnel: w458 -> [w460 _]
                                tunnel: [w460 w462] -> w457
                                tunnel: [w459 w461] -> w456
                                tunnel: w455 -> [w459 _]
                                tunnel: w454 -> [_ w462]
                                tunnel: w453 -> [_ w461]
                                frame False {
                                }
                                frame True {
                                }
                              }
                            }
                            frame True {
                            }
                          }
                        }
                        frame True {
                        }
                      }
                    }
                    frame True {
                    }
                  }
                  n153 = while {
                    tunnel: w428 -> [w482]
                    tunnel: [w479] -> w427
                    tunnel: w426 -> [w469]
                    tunnel: w421 -> [w470]
                    tunnel: w422 -> [w471]
                    i -> [w481]
                    stop <- w480 continue-if-true
                    n154 = File/Directory Info(path=w471) -> (error out=w473:errorcluster)  [unwired: 1 in, 6 out]
                    n155 = File/Directory Info(path=w470) -> (error out=w474:errorcluster)  [unwired: 1 in, 6 out]
                    n156 = Unbundle By Name(w473) -> ("status"=w477:bool)
                    n157 = Unbundle By Name(w474) -> ("status"=w478:bool)
                    n158 = Empty String/Path?(string/path=w470) -> (empty?=w476:bool)
                    n159 = Empty String/Path?(string/path=w471) -> (empty?=w475:bool)
                    n160 = Compound Arithmetic op=AND(invert w477, invert w475, invert w478, invert w476) -> (w472:bool)
                    n161 = case shown="True" w472 {
                      tunnel: w482 -> [w483 w495]
                      tunnel: w470 -> [_ w494]
                      tunnel: w471 -> [_ w493]
                      tunnel: w481 -> [_ w491]
                      tunnel: [_ w488] -> w480
                      tunnel: w469 -> [_ w487]
                      tunnel: [w483 w484] -> w479
                      frame False {
                      }
                      frame True {
                        n162 = Build Array(w493) -> (w486:path[])
                        n163 = Build Array(w494) -> (w485:path[])
                        n164 = call <resource>:"Scripting_ReplaceVisAndControls.vi"("ViRef"=w487, "OldVIsAndControls"=w486, "NewVIsAndControls"=w485, "error in (no error)"=w495) -> ("error out"=w484:errorcluster)  [unwired: 14 in, 1 out]
                        n165 = Unbundle By Name(w484) -> ("status"=w492:bool)  [unwired: 1 out]
                        n166 = Less Or Equal?(x=w491, y=3) -> (x <= y?=w489:bool)
                        n167 = And(x=w489, y=w492) -> (x .and. y?=w488:bool)
                      }
                    }
                  }
                }
              }
            }
            n168 = Unbundle By Name(w364) -> ("TempClass"=w363:refnum<vi>)
            n169 = stacked-sequence {
              tunnel: w363 -> [w378]
              tunnel: w362 -> [_]
              frame #0 {
                n170 = Close Reference(reference=w378) -> ()  [unwired: 1 in, 1 out]
              }
            }
          }
          frame "AnyProtectedAttributesToUpdate?" {
            n171 = Unbundle By Name(w497) -> ("BaseClassFolder"=w515:path)
            n172 = Unbundle By Name(w497) -> ("VIs"=w520:refnum<vi>[])
            n173 = call <vilib>:"Recursive File List.vi"("Folder Path"=w515) -> ("All Files in Dir"=w504:path[])  [unwired: 6 in, 4 out]
            n174 = for {
              tunnel: w520 -> [w548] mode=indexing
              tunnel: [w547] -> w501 mode=indexing
              tunnel: [w545] -> w517 mode=indexing
              n175 = property class="VI"(reference=w548) -> ("Path"=w547:path)  [unwired: 1 in, 2 out]
              n176 = Strip Path(path=w547) -> (name=w546:string)  [unwired: 1 out]
              n177 = To Lower Case(string=w546) -> (all lower case string=w545:string)
            }
            n178 = for {
              tunnel: w504 -> [w533] mode=indexing
              tunnel: [w532] -> w510 mode=indexing
              n179 = Strip Path(path=w533) -> (name=w534:string)  [unwired: 1 out]
              n180 = To Lower Case(string=w534) -> (all lower case string=w532:string)
            }
            n181 = To Lower Case(string="ObjectAttributes.ctl") -> (all lower case string=w514:string)
            n182 = Unbundle By Name(w497) -> ("App"=w496:refnum<vi>)
            n183 = To Lower Case(string="ClassAttributes.ctl") -> (all lower case string=w509:string)
            n184 = Search 1D Array(1D array=w510, element=w514) -> (index of element=w505:i32)  [unwired: 1 in]
            n185 = Search 1D Array(1D array=w510, element=w509) -> (index of element=w503:i32)  [unwired: 1 in]
            n186 = Search 1D Array(1D array=w517, element=w514) -> (index of element=w506:i32)  [unwired: 1 in]
            n187 = Search 1D Array(1D array=w517, element=w509) -> (index of element=w500:i32)  [unwired: 1 in]
            n188 = Greater Or Equal To 0?(x=w503) -> (x >= 0?=w508:bool)
            n189 = Greater Or Equal To 0?(x=w505) -> (x >= 0?=w512:bool)
            n190 = Greater Or Equal To 0?(x=w506) -> (x >= 0?=w513:bool)
            n191 = Greater Or Equal To 0?(x=w500) -> (x >= 0?=w507:bool)
            n192 = And(x=w512, y=w513) -> (x .and. y?=w511:bool)
            n193 = And(x=w508, y=w507) -> (x .and. y?=w502:bool)
            n194 = case shown="True" w511 {
              tunnel: w518 -> [w543 w544]
              tunnel: w501 -> [w542 _]
              tunnel: w504 -> [w540 _]
              tunnel: w506 -> [w538 _]
              tunnel: w505 -> [w537 _]
              tunnel: [w536 w544] -> w499
              tunnel: w496 -> [w535 _]
              frame True {
                n195 = Index Array(array=w542, index=w538) -> (element=w541:path)
                n196 = Index Array(array=w540, index=w537) -> (element=w539:path)
                n197 = call <resource>:"Scripting_UpdateProtectedClassData.vi"("AppRef"=w535, "error in (no error)"=w543, "NewBaseAttribute"=w539, "BaseAttribute"=w541) -> ("error out"=w536:errorcluster)  [unwired: 6 in, 1 out]
              }
              frame False {
              }
            }
            n198 = case shown="True" w502 {
              tunnel: w501 -> [w530 _]
              tunnel: w504 -> [w528 _]
              tunnel: w500 -> [w526 _]
              tunnel: w503 -> [w525 _]
              tunnel: w499 -> [w524 w531]
              tunnel: [w523 w531] -> w498
              tunnel: w496 -> [w522 _]
              frame True {
                n199 = Index Array(array=w530, index=w526) -> (element=w529:path)
                n200 = Index Array(array=w528, index=w525) -> (element=w527:path)
                n201 = call <resource>:"Scripting_UpdateProtectedClassData.vi"("AppRef"=w522, "error in (no error)"=w524, "NewBaseAttribute"=w527, "BaseAttribute"=w529) -> ("error out"=w523:errorcluster)  [unwired: 6 in, 1 out]
              }
              frame False {
              }
            }
          }
          frame "AddFolders" {
            n202 = Unbundle By Name(w550) -> ("ClassRefnum"=w563:refnum<vi>)
            n203 = Unbundle By Name(w550) -> ("TemplateName"=w562:string)
            n204 = call <resource>:"UpdateClassApperance.vi"("ClassRefIn"=w563, "error in (no error)"=w564) -> ("error out"=w557:errorcluster)  [unwired: 16 in, 1 out]
            n205 = call <resource>:"GOOP400_ConfigurationMemory.vi"("error in (no error)"=w557, "Action"=enum16{"Read", "Load", "Save"}."Read") -> ("OptionsOut"=w555:T13, "error out"=w556:errorcluster)  [unwired: 16 in]
            n206 = Unbundle By Name(w550) -> ("SubClass"=w551:bool)
            n207 = Unbundle By Name(w555) -> ("FlatFolderStructure"=w554:bool)
            n208 = Match Pattern(string=w562, regular expression="Interface") -> (offset past match=w560:i32)  [unwired: 1 in, 3 out]
            n209 = Greater Or Equal To 0?(x=w560) -> (x >= 0?=w559:bool)
            n210 = case shown="False" w559 {
              tunnel: [w571 w581] -> w565
              tunnel: w556 -> [w569 w581]
              tunnel: w563 -> [w568 _]
              tunnel: w554 -> [w567 _]
              frame False {
                (unwired) TRUE ("CreateThePfysicalFolderIfPossible(False)")
                n211 = Not(x=w567) -> (.not. x?=w566:bool)
                n212 = call <resource>:"GDSProject_CreateFolder.vi"("Project Item To Create Folder Below(Use MyComputer if not wired)"=w568, "FolderName"="private", "error in (no error)"=w569, "CreateThePhysicalFolderIfPossible(False)"=w566) -> ("ItemOut"=w574:refnum<vi>, "FolderCreated"=w570:bool, "error out"=w572:errorcluster)  [unwired: 12 in, 1 out]
                n213 = case shown="True" w570 {
                  tunnel: w574 -> [_ w576]
                  tunnel: w572 -> [w575 w579]
                  tunnel: [w575 w577] -> w571
                  tunnel: w568 -> [_ w578]
                  frame False {
                  }
                  frame True {
                    n214 = invoke class="LVClassLibrary" method="Set Source Scope"(reference=w578, error in=w579, "SourceRef"=w576, "Scope"=T8."private" ("scope")) -> (error out=w577:errorcluster)  [unwired: 1 in, 4 out]
                    n215 = Close Reference(reference=w576, error in (no error)=w577) -> ()  [unwired: 1 out]
                  }
                }
              }
              frame True {
              }
            }
            n216 = Select(t="ReplaceBaseTemplateReferences", s=w551, f="UpdateObjectRefEnum") -> (s? t:f=w549:string)
          }
          frame "UpdateObjectRefEnum" {
            w621 = refnum<vi> refnum  # Enum
            w624 = refnum<vi> refnum  # TypedRefNum
            n217 = Unbundle By Name(w583) -> ("App"=w586:refnum<vi>, "ClassFolder"=w587:path)
            n218 = Unbundle By Name(w583) -> ("ClassName"=w590:string)
            n219 = Build Path(base path=w587, name or relative path="ObjectReference.ctl") -> (appended path=w593:path)
            n220 = call <resource>:"Scripting_OpenViRef.vi"("error in"=w584, "ViPath/ViName/Viref"=w593, "AppRef"=w586) -> ("error out"=w605:errorcluster, "vi reference"=w606:refnum<vi>)  [unwired: 6 in, 1 out]
            n221 = invoke on="Save" class="VI" method="VI Icon.Get as Image Data"(reference=w606, error in=w605) -> (reference out=w604:refnum<vi>, error out=w603:errorcluster, "ImageData"=w602:T14)  [unwired: 4 in, 3 out]
            n222 = Unbundle By Name(w602) -> ("colors"=w599:u32[], "image"=w601:u8[])
            n223 = Delete From Array(array=w601, length=100, index=33) -> (deleted portion=w592:u8[])  [unwired: 1 out]
            n224 = property on="Panel" class="VI"(reference=w604, error in=w603) -> (reference out=w610:refnum<vi>, error out=w588:errorcluster, "Front Panel"=w589:refnum<vi>)
            n225 = property on="Ctrls" class="Pnl"(reference=w589, error in=w588) -> ("Controls[]"=w626:refnum<vi>[])  [unwired: 2 out]
            n226 = while {
              tunnel: w592 -> [w628] mode=indexing
              tunnel: [w628] -> w591
              i -> [w632]
              stop <- w629 continue-if-true
              w631 = 255
              n227 = Equal?(x=w628, y=w631) -> (x = y?=w633:bool)
              n228 = Less?(x=w632, y=w631) -> (x < y?=w630:bool)
              n229 = And(x=w633, y=w630) -> (x .and. y?=w629:bool)
            }
            n230 = Index Array(array=w626) -> (element=w625:refnum<vi>)  [unwired: 1 in]
            n231 = To More Specific Class(target class=w624, reference=w625, error in=w588) -> (specific class reference=w623:refnum<vi>, error out=w618:errorcluster)
            n232 = Build Array(w590) -> (w619:string[])
            n233 = property on="Ctrls" class="TypRef"(reference=w623, error in=w618) -> (reference out=w612:refnum<vi>, error out=w617:errorcluster, "Element"=w622:refnum<vi>)
            n234 = Index Array(array=w599, index=w591) -> (element=w596:u32)
            n235 = To More Specific Class(target class=w621, reference=w622, error in=w617) -> (specific class reference=w620:refnum<vi>, error out=w616:errorcluster)
            n236 = Equal To 0?(x=w596) -> (x = 0?=w597:bool)
            n237 = Select(t=u32 16777216, s=w597, f=w596) -> (s? t:f=w595:u32)
            n238 = property on="Ctrls" class="Enum"(reference=w620, error in=w616, "Strings []"=w619, "Named Numeric Colors:BG Color"=w595) -> (reference out=w615:refnum<vi>, error out=w614:errorcluster)
            n239 = Close Reference(reference=w615, error in (no error)=w614) -> (error out=w613:errorcluster)
            n240 = Close Reference(reference=w612, error in (no error)=w613) -> (error out=w611:errorcluster)
            n241 = Close Reference(reference=w589, error in (no error)=w611) -> (error out=w609:errorcluster)
            n242 = invoke on="Save" class="VI" method="Save.Instrument"(reference=w610, error in=w609) -> (reference out=w608:refnum<vi>, error out=w607:errorcluster)  [unwired: 4 in, 4 out]
            n243 = Close Reference(reference=w608, error in (no error)=w607) -> (error out=w585:errorcluster)
          }
          frame "ReplaceBaseTemplateReferences" {
            w643 = "ObjectReference.ctl" ("name or relative path")
            # "This is a sub class, replace all BaseClass References with Select base class.\nIf base not equal to root, also replace BaseClass ObjectRef with Root-Base ObjectRef"
            n244 = Unbundle By Name(w635) -> ("VIs"=w638:refnum<vi>[], "BaseClassFolder"=w636:path, "BaseClassName"=w637:string)  [unwired: 4 out]
            n245 = Unbundle By Name(w635) -> ("RootBaseClassFolder"=w651:path)
            n246 = Unbundle By Name(w635) -> ("TemplateParentName"=w650:string)
            n247 = call-dynamic "GetTemplatePath.vi"("reference in"=w641, "ClassTemplateSubDirectory"=w650) -> ("FolderPathOut"=w647:path)  [unwired: 13 in, 4 out]
            n248 = Build Path(base path=w647, name or relative path=w643) -> (appended path=w646:path)
            n249 = Build Path(base path=w651, name or relative path=w643) -> (appended path=w642:path)
            n250 = call <resource>:"GOOP300_FindFilesToExchange.vi"("OldClassName(Prefix or suffix for some VIs)"=w650, "OldFolderPath"=w647, "NewFolderPath"=w636, "NewClassName(Prefix or suffix for some VIs)"=w637) -> ("OldFiles"=w645:path[], "NewFileArray"=w644:path[])  [unwired: 14 in]
            n251 = Build Array (concatenate)(w646, w645) -> (w648:path[])
            n252 = Build Array (concatenate)(w642, w644) -> (w649:path[])
            n253 = for {
              tunnel: w638 -> [w656] mode=indexing
              shift-right: [w654] -> w640
              shift-left: w639 -> [w655]
              tunnel: w648 -> [w653]
              tunnel: w649 -> [w652]
              n254 = call <resource>:"Scripting_ReplaceVisAndControls.vi"("ViRef"=w656, "OldVIsAndControls"=w653, "NewVIsAndControls"=w652, "error in (no error)"=w655) -> ("error out"=w654:errorcluster)  [unwired: 14 in, 1 out]
            }
          }
          frame "PlaceRefInAttribute" {
            n255 = Unbundle By Name(w661) -> ("ClassRefnum"=w662:refnum<vi>)
            n256 = Unbundle By Name(w661) -> ("SubClass"=w658:bool, "RootBaseClassFolder"=w665:path)
            n257 = Unbundle By Name(w661) -> ("LvClassFolderPath"=w663:path)
            n258 = Select(t=w665, s=w658, f=w663) -> (s? t:f=w664:path)
            n259 = case shown="True" w658 {
              tunnel: w664 -> [_ w670]
              tunnel: w662 -> [_ w669]
              tunnel: w660 -> [w666 w668]
              tunnel: [w666 w667] -> w659
              frame False {
              }
              frame True {
                n260 = call <resource>:"Scripting_PlaceGoopRefInClassAttribute.vi"("error in"=w668, "ObjectRef_LvClassFolderPath"=w670, "ClassRefnum"=w669) -> ("error out"=w667:errorcluster)  [unwired: 1 in, 3 out]
              }
            }
          }
          frame "ReentrantDestructor?" {
            # "Use reentrant if this is a base class.\nor this is a sub class with a reentrant base class destructor"
            n261 = Unbundle By Name(w672) -> ("App"=w675:refnum<vi>, "BaseClassName"=w674:string, "VIs"=w676:refnum<vi>[])
            n262 = for {
              tunnel: w676 -> [w686] mode=indexing
              tunnel: w674 -> [w681]
              tunnel: w675 -> [w680]
              n263 = property class="VI"(reference=w686) -> (reference out=w682:refnum<vi>, "Name"=w685:string)  [unwired: 1 in, 1 out]
              n264 = Match Pattern(string=w685, regular expression=":Destroy\\2E[Vv][Ii]$") -> (offset past match=w683:i32)  [unwired: 1 in, 3 out]
              n265 = case shown="Default" w683 {
                tunnel: w682 -> [w691 _]
                tunnel: w681 -> [w690 _]
                tunnel: w680 -> [w687 _]
                frame Default {
                  n266 = case shown="\"False\", Default" w690 {
                    selector: w690 -> [w702 _]
                    tunnel: [w693 TRUE] -> w689
                    tunnel: w687 -> [w692 _]
                    frame "False", Default {
                      n267 = Concatenate Strings(w702, ".lvclass:Destroy.vi" ("regular expression")) -> (w700:string)
                      n268 = call <resource>:"Scripting_OpenViRef.vi"("ViPath/ViName/Viref"=w700, "AppRef"=w692) -> ("error out"=w698:errorcluster, "vi reference"=w699:refnum<vi>)  [unwired: 7 in, 1 out]
                      n269 = property class="VI"(reference=w699, error in=w698) -> (reference out=w697:refnum<vi>, error out=w696:errorcluster, "Exec.IsReentrant"=w694:bool)
                      n270 = Unbundle(w696) -> ("status"=w695:bool)  [unwired: 2 out]
                      n271 = Close Reference(reference=w697, error in (no error)=w696) -> ()  [unwired: 1 out]
                      n272 = Or(x=w695, y=w694) -> (x .or. y?=w693:bool)
                    }
                    frame "" {
                    }
                  }
                  n273 = property class="VI"(reference=w691, "Exec.IsReentrant"=w689, "Exec.ReentrancyType"=T9."Share clones between instances" ("Execution:Reentrancy Type")) -> ()  [unwired: 1 in, 2 out]
                }
                frame -1 {
                }
              }
            }
            n274 = Unbundle By Name(w672) -> ("llb"=w671:bool)
            n275 = case shown="False" w671 {
              tunnel: ["CloseRefs" "ConvertToLLb"] -> w677
              frame False {
              }
              frame True {
              }
            }
          }
          frame "ConvertToLLb" {
            n276 = Unbundle By Name(w720) -> ("ClassFolder"=w705:path)
            n277 = Unbundle By Name(w720) -> ("VIs"=w722:refnum<vi>[])
            n278 = Unbundle By Name(w720) -> ("ClassRefnum"=w719:refnum<vi>)
            n279 = Unbundle By Name(w725) -> ("ClassFolder"=w724:path)
            n280 = call <vilib>:"New VI Library.vi"("error in (no error)"=w723, "VI library path in"=w724) -> ("error out"=w721:errorcluster, "VI library path out"=w717:path)  [unwired: 8 in]
            n281 = for {
              tunnel: w722 -> [w739] mode=indexing
              tunnel: w717 -> [w736]
              shift-right: [w730] -> w707
              shift-left: w721 -> [w735]
              tunnel: w705 -> [w728]
              n282 = property class="VI"(reference=w739, error in=w735) -> (reference out=w738:refnum<vi>, error out=w734:errorcluster, "Path"=w737:path)
              n283 = Strip Path(path=w737) -> (stripped path=w729:path, name=w733:string)
              n284 = Build Path(base path=w736, name or relative path=w733) -> (appended path=w732:path)
              n285 = Equal?(x=w729, y=w728) -> (x = y?=w727:bool)
              n286 = invoke class="VI" method="Save.Instrument"(reference=w738, error in=w734, "Path to saved file"=w732) -> (error out=w731:errorcluster)  [unwired: 3 in, 5 out]
              n287 = case shown="True" w727 {
                tunnel: w732 -> [_ w744]
                tunnel: w731 -> [w740 w743]
                tunnel: [w740 w742] -> w730
                frame False {
                }
                frame True {
                  n288 = call <vilib>:"Librarian Get Info.vi"("error in (no error)"=w743, "path"=w744) -> ("error out"=w745:errorcluster, "file information"=w747:T15, "dup path"=w748:path)  [unwired: 7 in]
                  n289 = Bundle By Name(cluster=w747, "top level"=TRUE) -> (w746:T15)
                  n290 = call <vilib>:"Librarian Set Info.vi"("error in (no error)"=w745, "file information"=w746, "path"=w748) -> ("error out"=w742:errorcluster)  [unwired: 7 in, 1 out]
                }
              }
            }
            n291 = property class="LVClassLibrary"(reference=w719, error in=w707) -> (reference out=w715:refnum<vi>, "Path"=w718:path)  [unwired: 1 out]
            n292 = Strip Path(path=w718) -> (name=w716:string)  [unwired: 1 out]
            n293 = Build Path(base path=w717, name or relative path=w716) -> (appended path=w709:path)
            n294 = invoke class="LVClassLibrary" method="Save"(reference=w715, "Path"=w709) -> (error out=w708:errorcluster)  [unwired: 2 in, 3 out]
            n295 = call <vilib>:"Librarian Get Info.vi"("error in (no error)"=w708, "path"=w709) -> ("error out"=w713:errorcluster, "file information"=w711:T15, "dup path"=w710:path)  [unwired: 7 in]
            n296 = Bundle By Name(cluster=w711, "top level"=TRUE) -> (w712:T15)
            n297 = call <vilib>:"Librarian Set Info.vi"("error in (no error)"=w713, "file information"=w712, "path"=w710) -> ("error out"=w706:errorcluster)  [unwired: 7 in, 1 out]
            n298 = Delete(path (use dialog)=w705, entire hierarchy (F)=TRUE, error in=w706) -> ()  [unwired: 2 in, 3 out]
          }
          frame "CloseRefs", "Error", Default {
            n299 = case shown="\"CloseRefs\"" w767 {
              tunnel: w768 -> [w790 w798]
              tunnel: w751 -> [w789 w794]
              tunnel: [w790 w797] -> w752
              frame "False", Default {
                n300 = Unbundle By Name(w789) -> ("VIs"=w788:refnum<vi>[])
                n301 = Close Reference(reference=w788) -> ()  [unwired: 1 in, 1 out]
              }
              frame "CloseRefs" {
                n302 = Unbundle By Name(w794) -> ("ClassRefnum"=w793:refnum<vi>)
                n303 = Unbundle By Name(w794) -> ("ViLocked"=w796:bool[], "VIs"=w799:refnum<vi>[])
                n304 = Unbundle By Name(w794) -> ("ClassSettings"=w795:T2)
                n305 = call <resource>:"GDSLvClass_StoreClassType.vi"("Class Refnum In"=w793, "ClassSettings"=w795, "CheckAndFixConnectorPaneType(False)"=TRUE) -> ("error out"=w791:errorcluster)  [unwired: 15 in, 1 out]
                n306 = for {
                  tunnel: w799 -> [w804] mode=indexing
                  shift-right: [w800] -> w797
                  shift-left: w798 -> [w805]
                  tunnel: w796 -> [w801] mode=indexing
                  tunnel: w791 -> [_]
                  n307 = case shown="True" w801 {
                    tunnel: w805 -> [w809 w815]
                    tunnel: w804 -> [w810 w814]
                    tunnel: [w809 w813] -> w803
                    tunnel: [w810 w812] -> w802
                    frame False {
                    }
                    frame True {
                      n308 = invoke class="VI" method="Lock State.Set"(reference=w814, error in=w815, "lockState"=T10."Locked (No Password)" ("Lock State")) -> (reference out=w812:refnum<vi>, error out=w813:errorcluster)  [unwired: 4 in, 5 out]
                    }
                  }
                  n309 = call <resource>:"Scripting_SaveVi.vi"("ForceResaving(False)"=TRUE, "error in (no error)"=w803, "VIRefToSaveIn"=w802) -> ("error out"=w808:errorcluster, "VIRefToSaveOut"=w807:refnum<vi>)  [unwired: 7 in]
                  n310 = Close Reference(reference=w807, error in (no error)=w808) -> (error out=w800:errorcluster)
                }
              }
            }
            n311 = Unbundle By Name(w751) -> ("TempClass"=w750:refnum<vi>)
            n312 = stacked-sequence {
              tunnel: w752 -> [w770]
              tunnel: [w770] -> w749
              tunnel: w750 -> [w771]
              frame #0 {
                n313 = Close Reference(reference=w771) -> ()  [unwired: 1 in, 1 out]
              }
            }
            n314 = Unbundle By Name(w751) -> ("DeleteFiles"=w762:path[], "App"=w754:refnum<vi>, "ProjectRefnum"=w765:refnum<vi>, "ClassRefnum"=w761:refnum<vi>)
            n315 = call <resource>:"GDSLvClass_SaveEverythingInClass.vi"("ClassRefIn"=w761, "error in"=w749) -> ("ClassRefOut"=w756:refnum<vi>, "error out"=w758:errorcluster)  [unwired: 16 in]
            n316 = case shown="False" w759 {
              tunnel: [w774 w775] -> w766
              tunnel: w758 -> [w773 w775]
              tunnel: w756 -> [w772 _]
              frame False {
                n317 = Close Reference(reference=w772, error in (no error)=w773) -> (error out=w774:errorcluster)
              }
              frame True {
              }
            }
            n318 = Close Reference(reference=w765, error in (no error)=w766) -> (error out=w755:errorcluster)
            n319 = Close Reference(reference=w754, error in (no error)=w755) -> (error out=w753:errorcluster)
            n320 = for {
              shift-right: [w786] -> w757
              shift-left: w753 -> [w787]
              tunnel: w762 -> [w785] mode=indexing
              tunnel: [w784] -> w760 mode=indexing
              n321 = Delete(path (use dialog)=w785, error in=w787) -> (error out=w786:errorcluster)  [unwired: 3 in, 2 out]
              n322 = Strip Path(path=w785) -> (stripped path=w784:path)  [unwired: 1 out]
            }
            n323 = for {
              tunnel: w760 -> [w780] mode=indexing
              n324 = List Folder(path=w780) -> (path out=w776:path, filenames=w779:string[], error out=w777:errorcluster)  [unwired: 3 in, 1 out]
              n325 = Empty Array?(array=w779) -> (empty?=w778:bool)
              n326 = case shown="True" w778 {
                tunnel: w777 -> [_ w783]
                tunnel: w776 -> [_ w782]
                tunnel: [_ w781] -> _
                frame False {
                }
                frame True {
                  n327 = Delete(path (use dialog)=w782, error in=w783) -> (error out=w781:errorcluster)  [unwired: 3 in, 2 out]
                }
              }
            }
            n328 = call <resource>:"GDSError_LogErrorInformation.vi"("State"=w763, "LocalVariableData"=w751, "error in (no error)"=w757) -> ("error out"=w764:errorcluster)  [unwired: 16 in]
          }
        }
        n329 = Equal?(x=w34, y="Exit") -> (x = y?=w38:bool)
        n330 = Select(t="Error", s=w33, f=w34) -> (s? t:f=w37:string)
      }
      n331 = Unbundle By Name(w14) -> ("ClassRefnum"=w17:refnum<vi>, "TemplateVersion"=w16:string)
    }
    frame Error {
    }
  }
  "error out" <- w11
  "LVClassLibraryRefnum" <- w5
  "TemplateVersionUsed" <- w4
  "ClassWriterGOOP300.lvclass" <- "ClassWriterGOOP300.lvclass"
